vi "Initialize With Dialog.vi"(8 "error in (no error)":errorcluster, 11 "Sound Player in":refnum<class "Sound Visualizer.lvclass">) -> (0 "error out":errorcluster, 2 "Cancelled?":bool, 3 "Sound Player out":refnum<class "Sound Visualizer.lvclass">)   [LabVIEW 2010, in "Sound Visualizer.lvclass"]
doc: "Show configuration dialog for the Visualizer."
uses:
  Sound Visualizer.lvclass
  <vilib>/Utility/miscctls.llb/LVRectTypeDef.ctl
  Sound Visualizer.lvclass/Sound Visualizer.ctl
  Visualizer/Visualizer.lvlib
panel:
  in  "Select colors for plot:":u32[](array[colorbox])=[16777215, 16711680]
  in  "custom bounds?":bool
  in  "Front Panel Bounds":T1={"Left"=0, "Top"=0, "Right"=360, "Bottom"=216} {"Right" min=360 max=1024; "Bottom" min=216 max=768}
  in  "Cancel":bool
  in  "OK":bool
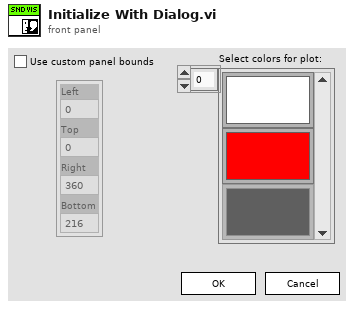
[diagram p1: front panel]
types:
  T1 = typedef "LVRectTypeDef.ctl" = cluster{"Left":i16, "Top":i16, "Right":i16, "Bottom":i16}
  T2 = enum8{"Enabled", "Disabled", "Disabled and Grayed Out"}
  T3 = typedef "Visualizer.lvlib/Visualizer Type ID.ctl" = u32
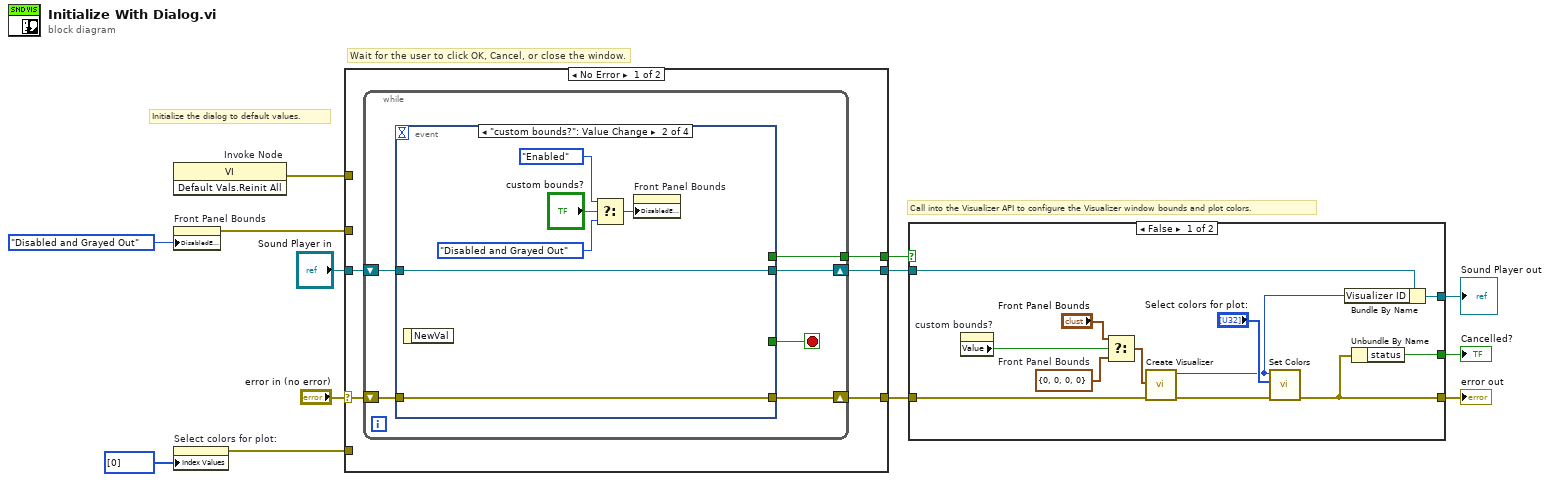
[diagram p0: block diagram]
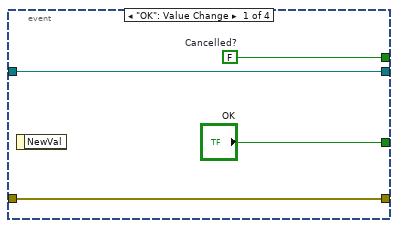
[diagram p3: hidden frame]
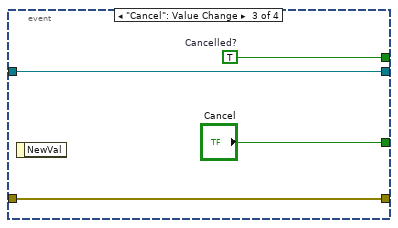
[diagram p4: hidden frame]
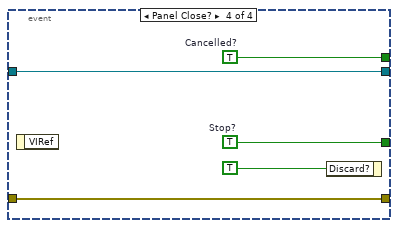
[diagram p5: hidden frame]
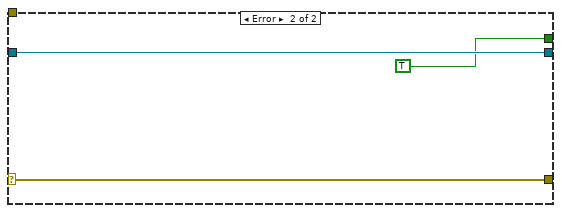
[diagram p6: hidden frame]
diagram:
  # "Call into the Visualizer API to configure the Visualizer window bounds and plot colors."
  # "Wait for the user to click OK, Cancel, or close the window."
  # "Initialize the dialog to default values."
  n1 = invoke on="Invoke Node" class="VI" method="Default Vals.Reinit All"() -> (error out=w1:errorcluster)  [unwired: 3 in, 2 out]
  n2 = property on="Front Panel Bounds" class="Clust (strict)"("DisabledEnum"=T2."Disabled and Grayed Out" ("Disabled")) -> (error out=w10:errorcluster)  [unwired: 2 in, 1 out]
  n3 = property on="Select colors for plot:" class="Arr (strict)"("Index Values"=u32[] [0]) -> (error out=w2:errorcluster)  [unwired: 2 in, 1 out]
  n4 = case shown="No Error" "error in (no error)" {
    selector: "error in (no error)" -> [w16 w46]
    tunnel: [w18 TRUE ("Cancelled?")] -> w9
    tunnel: [w15 w46] -> w7
    tunnel: [w17 w45] -> w8
    tunnel: "Sound Player in" -> [w14 w45]
    tunnel: w10 -> [_ _]
    tunnel: w2 -> [_ _]
    tunnel: w1 -> [_ _]
    frame No Error {
      n5 = while {
        tunnel: [w23] -> w18
        shift-right: [w22] -> w17
        shift-left: w14 -> [w21]
        shift-right: [w19] -> w15
        shift-left: w16 -> [w20]
        stop <- w24 stop-if-true
        n6 = event shown="[1] \"custom bounds?\": Value Change" {
          selector: _ -> [_ _ _ _]
          dyn-events: _ -> [_ _ _ _]
          timeout: _ -> [_ _ _ _]
          tunnel: ["OK" _ "Cancel" w42] -> w24
          tunnel: [w28 _ w38 w41] -> w23
          tunnel: [w26 w34 w36 w40] -> w22
          tunnel: w21 -> [w26 w34 w36 w40]
          tunnel: w20 -> [w25 w33 w35 w39]
          tunnel: [w25 w33 w35 w39] -> w19
          event "OK": Value Change {
            w28 = FALSE  # Cancelled?
            n7 = event-data() -> ()  [unwired: 1 in, 1 out]
          }
          event "custom bounds?": Value Change {
            n8 = event-data() -> ()  [unwired: 1 in, 1 out]
            n9 = Select(t=T2."Enabled" ("Disabled"), s="custom bounds?", f=T2."Disabled and Grayed Out" ("Disabled")) -> (s? t:f=w29:T2)
            n10 = property on="Front Panel Bounds" class="Clust (strict)"("DisabledEnum"=w29) -> ()  [unwired: 2 in, 2 out]
          }
          event "Cancel": Value Change {
            w38 = TRUE  # Cancelled?
            n11 = event-data() -> ()  [unwired: 1 in, 1 out]
          }
          event Panel Close? {
            w41 = TRUE  # Cancelled?
            w42 = TRUE  # Stop?
            n12 = event-data() -> ()  [unwired: 1 in, 1 out]
            n13 = event-data("Discard?"=TRUE) -> ()  [unwired: 1 in, 1 out]
          }
        }
      }
    }
    frame Error {
    }
  }
  n14 = case shown="False" w9 {
    selector: w9 -> [_ w60]
    tunnel: w8 -> [w51 w61]
    tunnel: w7 -> [w54 w59]
    tunnel: [w49 w61] -> w6
    tunnel: [w48 w59] -> w5
    tunnel: [w47 w60] -> w4
    frame False {
      w56 = T1 {"Left"=0, "Top"=0, "Right"=0, "Bottom"=0}  # Front Panel Bounds
      n15 = property on="custom bounds?" class="Bool (strict)"() -> ("Value"=w58:bool)  [unwired: 2 in, 2 out]
      n16 = Select(t="Front Panel Bounds", s=w58, f=w56) -> (s? t:f=w55:T1)
      n17 = call "Create Visualizer.vi"("error in (no error)"=w54, "Front Panel Bounds"=w55) -> ("error out"=w53:errorcluster, "Visualizer ID"=w50:T3)  [unwired: 8 in]
      n18 = call "Set Colors.vi"("error in (no error)"=w53, "Colors"="Select colors for plot:", "Visualizer ID"=w50) -> ("error out"=w48:errorcluster)  [unwired: 8 in]
      n19 = Bundle By Name(cluster=w51, "Visualizer ID"=w50) -> (w49:refnum<class "Sound Visualizer.lvclass">)
      n20 = Unbundle By Name(w48) -> ("status"=w47:bool)
    }
    frame True {
    }
  }
  "Cancelled?" <- w4
  "error out" <- w5
  "Sound Player out" <- w6
